vi "Stop Core.vi"(10 "final error code":i32, 11 "Controller Actor In":refnum<class "Controller Actor.lvclass">) -> (3 "Controller Actor Out":refnum<class "Controller Actor.lvclass">)   [LabVIEW 2016, in "Event Actors.lvlib" / "Controller Actor.lvclass"]
doc: "(<B>Filename</B>: Actor Framework.lvlib:Actor.lvclass:Stop Core.vi)\n\nDefines what the actor does before it stops. Use the <B>final error code</B> input to determine whether the actor shut down in response to an error.\n\nBy default, this method does nothing. A descendant class may override it to define behavior, such as shutting down any processes the actor initiated in its override of the Actor Core method."
uses:
  Controller Actor.lvclass
  Controller Actor.lvclass/Controller Actor.ctl
  <vilib>/MGI/Monitored Actor/Monitored Actor/Monitored Actor/Monitored Actor.lvclass
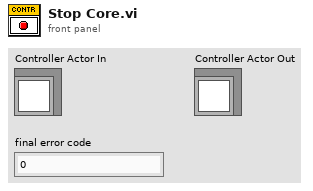
[diagram p1: front panel]
types:
  T1 = typedef "Event Actors.lvlib/Controller Actor.lvclass/View Settings Event Ref.ctl" = refnum<user-event>
  T2 = typedef "Event Actors.lvlib/Controller Actor.lvclass/Registered Views Event Ref.ctl" = refnum<user-event>
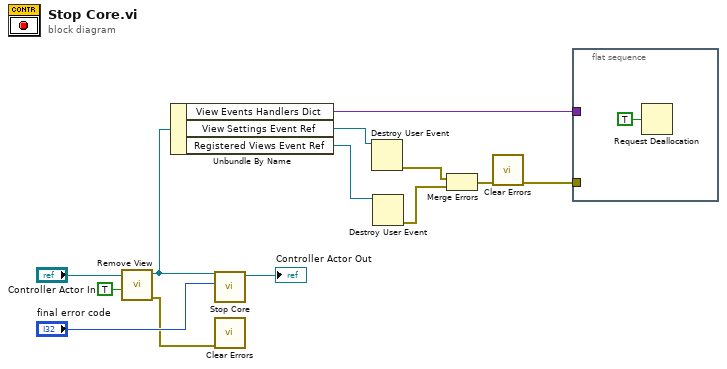
[diagram p0: block diagram]
diagram:
  n1 = call "Remove View.vi"("Remove All (F)"=TRUE, "Controller Actor in"="Controller Actor In") -> ("error out"=w7:errorcluster, "Controller Actor out"=w9:refnum<class "Controller Actor.lvclass">)  [unwired: 8 in]
  n2 = Unbundle By Name(w9) -> ("View Events Handlers Dict"=w11:variant, "View Settings Event Ref"=w6:T1, "Registered Views Event Ref"=w5:T2)
  n3 = call-parent "Stop Core.vi"("final error code"="final error code", "Monitored Actor in"=w9) -> ("Monitored Actor out"=→"Controller Actor Out":refnum<class "Controller Actor.lvclass">)  [unwired: 9 in]
  n4 = call <vilib>:"Clear Errors.vi"("error in (no error)"=w7) -> ()  [unwired: 5 in, 2 out]
  n5 = Destroy User Event(user event=w6) -> (error out=w3:errorcluster)  [unwired: 1 in]
  n6 = Destroy User Event(user event=w5) -> (error out=w2:errorcluster)  [unwired: 1 in]
  n7 = Merge Errors(w3, w2) -> (w4:errorcluster)
  n8 = call <vilib>:"Clear Errors.vi"("error in (no error)"=w4) -> ("error out"=w1:errorcluster)  [unwired: 5 in, 1 out]
  n9 = flat-sequence {
    tunnel: w11 -> [_]
    tunnel: w1 -> [_]
    frame #0 {
      n10 = Request Deallocation(TRUE ("flag")) -> ()
    }
  }
